vi "Get OFDM Data Rate (Mbps).vi"(8 "error in (no error)":errorcluster, 11 "niDTS WLAN Dut in":refnum<class "niDTS WLAN Dut.lvclass">) -> (0 "error out":errorcluster, 2 "OFDM Data Rate (Mbps)":T1, 3 "niDTS WLAN Dut out":refnum<class "niDTS WLAN Dut.lvclass">)   [LabVIEW 2015, in "niDTS WLAN.lvlib" / "niDTS WLAN Dut.lvclass"]
uses:
  niDTS WLAN Dut.lvclass
  Includes/niDTS WLAN INC OFDM Data Rate.ctl
  niDTS WLAN Dut.lvclass/niDTS WLAN Dut.ctl
  niDTS WLAN.lvlib
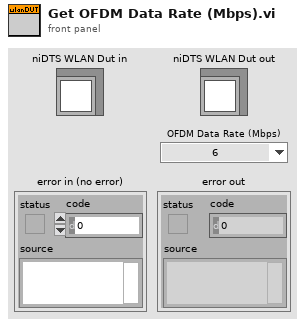
[diagram p1: front panel]
types:
  T1 = typedef "niDTS WLAN.lvlib/niDTS WLAN INC OFDM Data Rate.ctl" = enum16{"6", "9", "12", "18", "24", "36", "48", "54"}
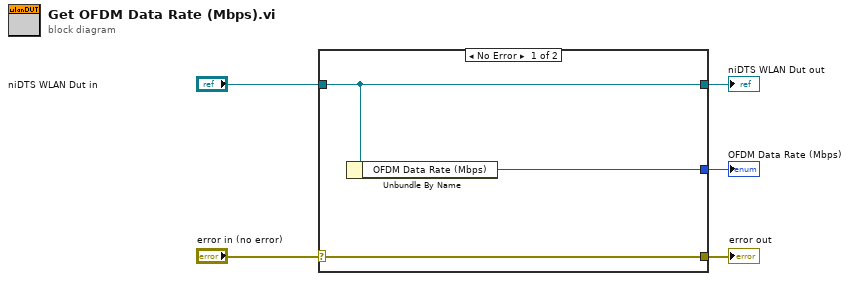
[diagram p0: block diagram]
diagram:
  n1 = case shown="No Error" "error in (no error)" {
    selector: "error in (no error)" -> [w8 w9]
    tunnel: [w8 w9] -> w4
    tunnel: [w7 w10] -> w2
    tunnel: "niDTS WLAN Dut in" -> [w7 w10]
    tunnel: [w6 _] -> w1
    frame No Error {
      n2 = Unbundle By Name(w7) -> ("OFDM Data Rate (Mbps)"=w6:T1)
    }
    frame Error {
    }
  }
  "error out" <- w4
  "niDTS WLAN Dut out" <- w2
  "OFDM Data Rate (Mbps)" <- w1
